vi "LongpressButton.vi"(2 "Threshold (ms)":u32=100, 3 "Button":bool) -> (0 "Starting Press":bool, 1 "Longpress Button":bool)   [LabVIEW 2019]
doc: "This VI takes as input a Boolean button press, and only returns TRUE if the button has been held continuously for longer than the specified time threshold."
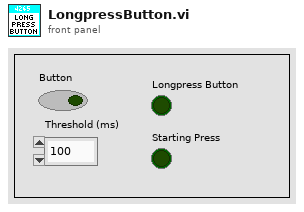
[diagram p1: front panel]
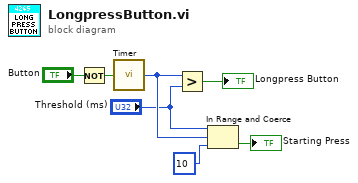
[diagram p0: block diagram]
diagram:
  n1 = Not(x="Button") -> (.not. x?=w6:bool)
  n2 = call "Timer.vi"("Reset Timer"=w6) -> ("Time (ms)"=w4:u32)
  n3 = Greater?(x=w4, y="Threshold (ms)") -> (0:→"Longpress Button":bool)
  n4 = In Range and Coerce(upper limit="Threshold (ms)", x=w4, lower limit=u32 10) -> (In Range?=→"Starting Press":bool)  [unwired: 1 out]
